vi "Logger_Create.vi"(0 "reference in":refnum<class "Logger.lvclass">, 5 "error in (no error)":errorcluster, 6 "DatabaseInterface":refnum<class "DatabaseInterface.lvclass">) -> (14 "reference out":refnum<class "Logger.lvclass">, 19 "error out":errorcluster)   [LabVIEW 2019, in "Logger.lvclass"]
doc: "Constructor."
uses:
  Logger.lvclass
  DatabaseInterface_class/DatabaseInterface.lvclass
  SignalData.ctl
  ObjData.ctl
  ObjType.ctl
  EventData.ctl
  TypeDef/AlarmType.ctl
  Logger.lvclass/Logger.ctl
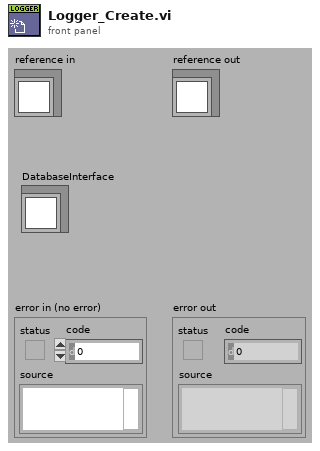
[diagram p1: front panel]
types:
  T1 = typedef "Logger.lvclass/SignalData.ctl" = cluster{"Value":dbl, "SignalTag":string, "ObjTag":string, "Desc":string, "Time Stamp":timestamp}
  T2 = typedef "Logger.lvclass/ObjData.ctl" = cluster{"object_tag":string, "parent_tag":string, "object_type":T3, "description":string}
  T3 = typedef "Logger.lvclass/ObjType.ctl" = enum16{"Procces", "Device", "Signal", "DI", "DO", "DA", "AI", "AO", "AA"}
  T4 = typedef "EventData.ctl" = cluster{"obj_tag":string, "event_tag":string, "Description":string, "ALARM TYPE":T5, "Value DBL":dbl, "Value INT":i32, "Value STR":string, "Time Stamp":timestamp}
  T5 = typedef "AlarmType.ctl" = enum16{"Normal", "Warning", "Alarm"}
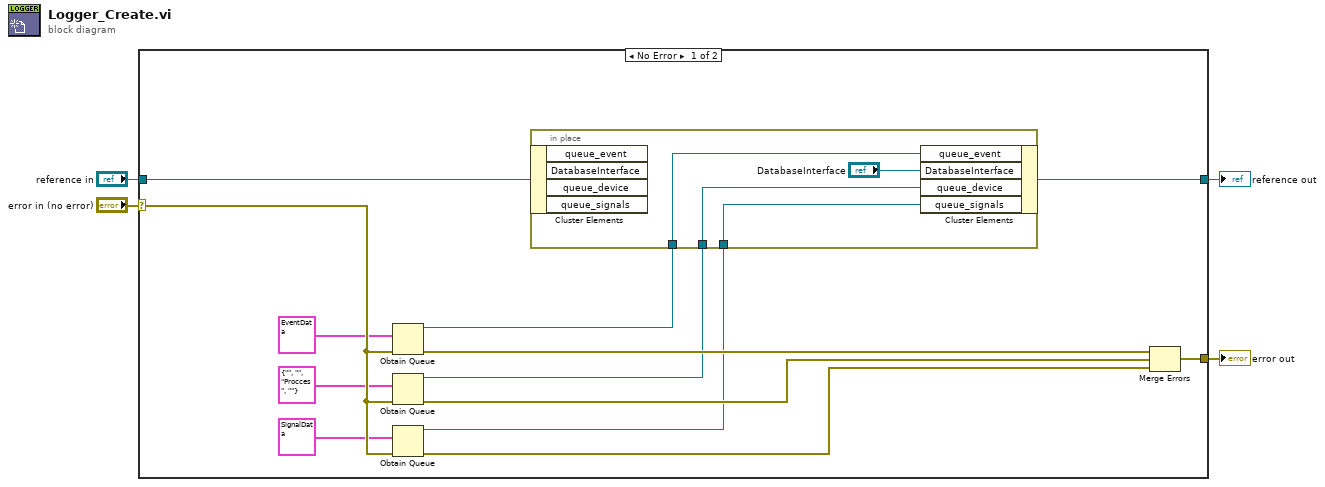
[diagram p0: block diagram]
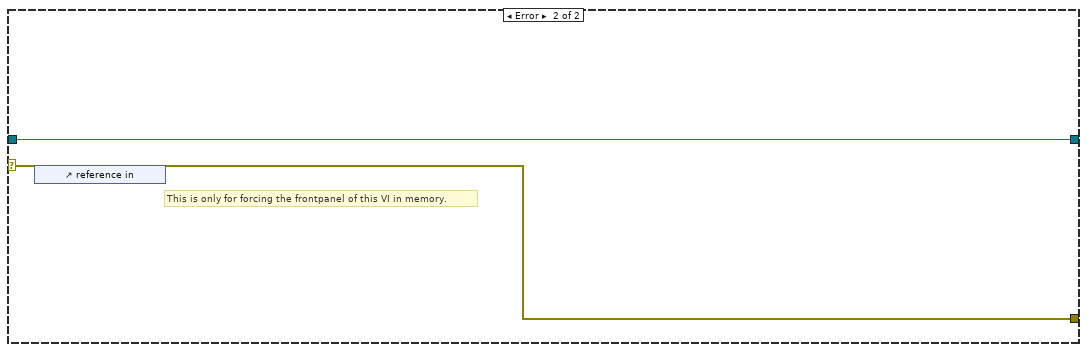
[diagram p2: hidden frame]
diagram:
  n1 = case shown="No Error" "error in (no error)" {
    selector: "error in (no error)" -> [w17 w23]
    tunnel: [w16 w23] -> w3
    tunnel: [w6 w22] -> w1
    tunnel: "reference in" -> [w5 w22]
    frame No Error {
      n2 = Obtain Queue(element data type=T4 {"obj_tag"="", "event_tag"="", "Description"="", "ALARM TYPE"=enum."Alarm", "Value DBL"=0.0, "Value INT"=0, "Value STR"="", "Time Stamp"=timestamp(0 s since 1904-01-01)} ("Event"), error in (no error)=w17) -> (queue out=w13:refnum<queue>, error out=w15:errorcluster)  [unwired: 3 in, 1 out]
      n3 = Obtain Queue(element data type=T2 {"object_tag"="", "parent_tag"="", "object_type"=enum."Procces", "description"=""} ("ObjData"), error in (no error)=w17) -> (queue out=w11:refnum<queue>, error out=w10:errorcluster)  [unwired: 3 in, 1 out]
      n4 = Obtain Queue(element data type=T1 {"Value"=0.0, "SignalTag"="", "ObjTag"="", "Desc"="", "Time Stamp"=timestamp(0 s since 1904-01-01)} ("SignalData"), error in (no error)=w17) -> (queue out=w8:refnum<queue>, error out=w7:errorcluster)  [unwired: 3 in, 1 out]
      n5 = in-place {
        in-place-border: w13 -> [w21]
        in-place-border: w11 -> [w19]
        in-place-border: w8 -> [w18]
        n6 = in-place-cluster #1(w5) -> ()  [unwired: 4 out]
        n7 = in-place-cluster #1("queue_event"=w21, "DatabaseInterface"="DatabaseInterface", "queue_device"=w19, "queue_signals"=w18) -> (w6:refnum<class "Logger.lvclass">)
      }
      n8 = Merge Errors(w15, w10, w7) -> (w16:errorcluster)
    }
    frame Error {
      # "This is only for forcing the frontpanel of this VI in memory."
      n9 = control-ref of="reference in"() -> ()  [unwired: 1 out]
    }
  }
  "error out" <- w3
  "reference out" <- w1
